vi "load_external_coordinates_grMD.vi"() -> ()   [LabVIEW 2017]
doc: "SciScan 1.2 160622"
uses:
  GFG/GFGDisplayRefsGet.vi
  GFG/GFGfpRefGet.vi
  GFG/GFGImageRefsGet.vi
  <vilib>/Utility/file.llb/Read From Spreadsheet File (I64).vi
  GFG/GFG library.lvlib
panel:
  out "error out":errorcluster
  in  "error in (no error)":errorcluster
  in  "stop":bool
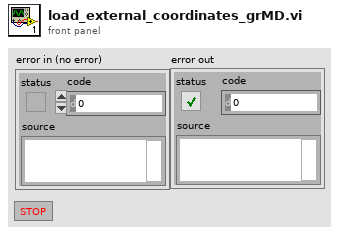
[diagram p1: front panel]
types:
  T1 = cluster{"Channel 1 small":refnum<vi>, "Channel 2 small":refnum<vi>, "Channel 3 small":refnum<vi>, "Channel 4 small":refnum<vi>, "Channel 1 large":refnum<vi>, "Channel 2 large":refnum<vi>, "Channel 3 large":refnum<vi>, "Channel 4 large":refnum<vi>, "RGB overlay":refnum<vi>, "ROI Image display":refnum<vi>, "arb line scan display":refnum<vi>, "Channel 5 large":refnum<vi>}
  T2 = typedef "IMAQ Image.ctl" = refnum<image>
  T3 = cluster{"Channel 1 small":T2, "Channel 2 small":T2, "Channel 3 small":T2, "Channel 4 small":T2, "Channel 1 large":T2, "Channel 2 large":T2, "Channel 3 large":T2, "Channel 4 large":T2, "RGB overlay":T2, "ROI Image display":T2, "arb line scan display":T2, "Channel 5 large":T2}
  T4 = cluster{"Contour Type":u32, "ROI Type":u32, i32[]}
  T5 = cluster{"Contour Type":u32, "ROI Type":u32, i32[]}[]
  T6 = cluster{i32[], cluster{"Contour Type":u32, "ROI Type":u32, i32[]}[]}
  T7 = cluster{"WaveformChartRef":refnum<vi>, "DigitalRef":refnum<vi>, "ArrayRef":refnum<vi>, "TabControlRef":refnum<vi>, "EnumRef":refnum<vi>, "RingRef":refnum<vi>, "BooleanRef":refnum<vi>, "KnobRef":refnum<vi>, "SlideRef":refnum<vi>, "PathRef":refnum<vi>, "StringRef":refnum<vi>, "ComboBox":refnum<vi>, "WaveformGraphRef":refnum<vi>}
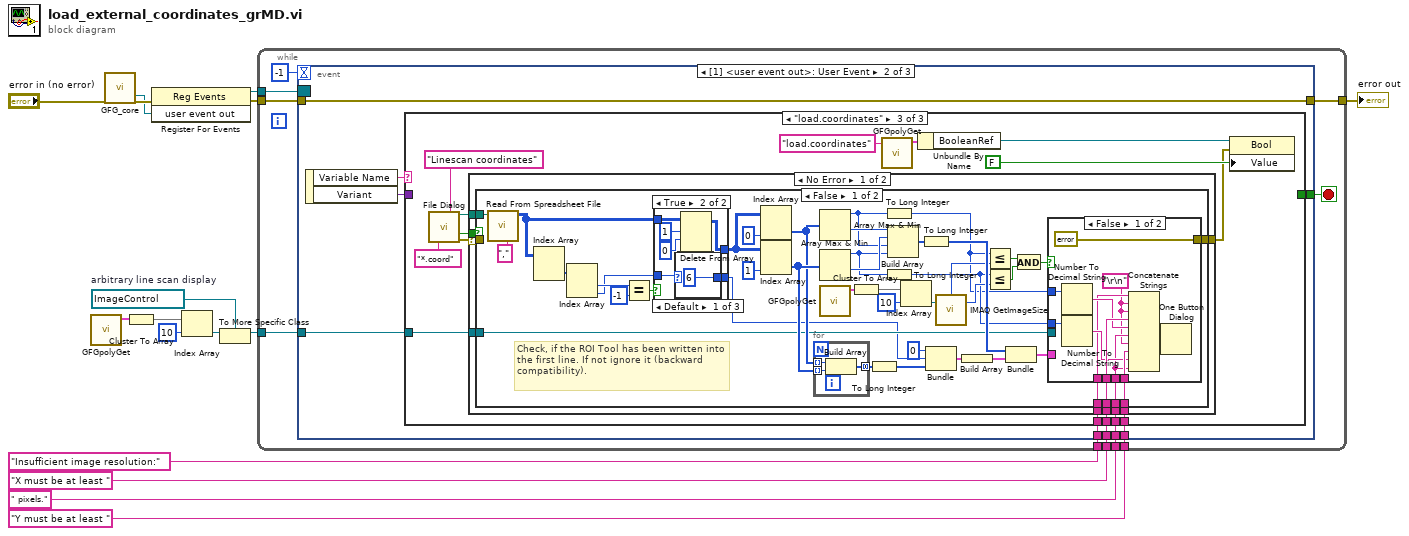
[diagram p0: block diagram]
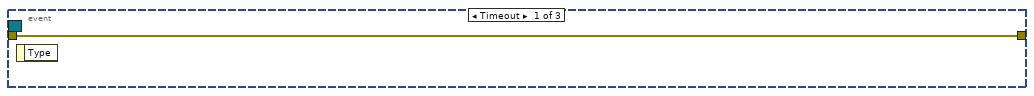
[diagram p2: hidden frame]
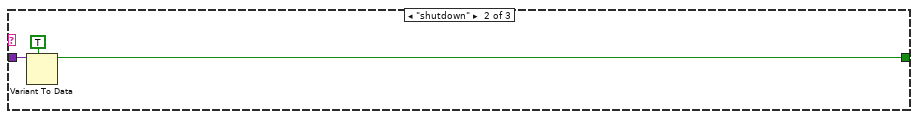
[diagram p4: hidden frame]
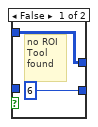
[diagram p5: hidden frame]
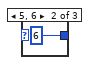
[diagram p6: hidden frame]
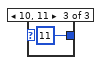
[diagram p7: hidden frame]
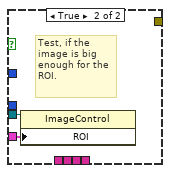
[diagram p8: hidden frame]
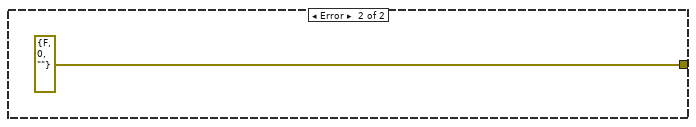
[diagram p10: hidden frame]
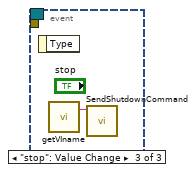
[diagram p11: hidden frame]
diagram:
  w16 = refnum<vi> refnum  # arbitrary line scan display
  n1 = call-poly "GFGpolyGet.vi"() -> ("DisplayRefsOut(generic class)"=w15:T1)  [unwired: 10 in, 1 out]
  n2 = call "GFG_core.vi"("error in (no error)"="error in (no error)") -> ("user event out"=w10:refnum<user-event>, "error out"=w11:errorcluster)  [unwired: 12 in, 5 out]
  n3 = Cluster To Array(cluster=w15) -> (array=w7:refnum<vi>[])
  n4 = register-events(error in=w11, w10) -> (reference out=w9:refnum<event-registration>, error out=w13:errorcluster)  [unwired: 1 in]
  n5 = Index Array(array=w7, index=10) -> (element=w5:refnum<vi>)
  n6 = To More Specific Class(target class=w16, reference=w5) -> (specific class reference=w8:refnum<vi>)  [unwired: 1 in, 1 out]
  n7 = while {
    tunnel: w9 -> [w26]
    tunnel: w13 -> [w24]
    tunnel: [w23] -> w14
    tunnel: w8 -> [w21]
    tunnel: "Insufficient image resolution:" ("message") -> [w20]
    tunnel: "X must be at least " ("message") -> [w19]
    tunnel: " pixels." ("message") -> [w18]
    tunnel: "Y must be at least " ("message") -> [w17]
    stop <- w25 stop-if-true
    n8 = event shown="[1] <user event out>: User Event" {
      selector: w26 -> [_ _ _]
      dyn-events: _ -> [_ _ _]
      timeout: -1 -> [_ _ _]
      tunnel: [_ w35 _] -> w25
      tunnel: w24 -> [w27 w34 _]
      tunnel: [w27 w34 _] -> w23
      tunnel: w21 -> [_ w33 _]
      tunnel: w20 -> [_ w31 _]
      tunnel: w19 -> [_ w30 _]
      tunnel: w18 -> [_ w29 _]
      tunnel: w17 -> [_ w28 _]
      event Timeout {
        n9 = event-data() -> ()  [unwired: 1 in, 1 out]
      }
      event User Event {
        n10 = event-data() -> ("Variable Name"=w36:string, "Variant"=w32:variant)  [unwired: 1 in]
        n11 = case shown="\"load.coordinates\"" w36 {
          tunnel: w32 -> [_ w39 _]
          tunnel: [_ w37 _] -> w35
          tunnel: w33 -> [_ _ w54]
          tunnel: w31 -> [_ _ w43]
          tunnel: w30 -> [_ _ w42]
          tunnel: w29 -> [_ _ w41]
          tunnel: w28 -> [_ _ w40]
          frame Default {
          }
          frame "shutdown" {
            n12 = Variant To Data(type=TRUE ("want seconds? (F)"), Variant=w39) -> (data=w37:bool)  [unwired: 1 in, 1 out]
          }
          frame "load.coordinates" {
            n13 = call "File Dialog"("pattern (all files)"="*.coord", "pattern label"="Linescan coordinates" ("pattern (all files)")) -> ("selected path"=w53:path, "cancelled"=w46:bool, "error out"=w52:errorcluster)  [unwired: 10 in, 1 out]
            n14 = case shown="No Error" w52 {
              selector: w52 -> [w60 _]
              tunnel: w54 -> [w63 _]
              tunnel: w53 -> [w62 _]
              tunnel: w46 -> [w61 _]
              tunnel: [w59 errorcluster {"status"=FALSE, "code"=0, "source"=""} ("error out")] -> w45
              tunnel: w43 -> [w58 _]
              tunnel: w42 -> [w57 _]
              tunnel: w41 -> [w56 _]
              tunnel: w40 -> [w55 _]
              frame No Error {
                n15 = case shown="False" w61 {
                  tunnel: w63 -> [w91 _]
                  tunnel: w62 -> [w90 _]
                  tunnel: w60 -> [_ _]
                  tunnel: [w81 _] -> w59
                  tunnel: w58 -> [w75 _]
                  tunnel: w57 -> [w74 _]
                  tunnel: w56 -> [w73 _]
                  tunnel: w55 -> [w72 _]
                  frame False {
                    # "Check, if the ROI Tool has been written into the first line. If not ignore it (backward compatibility)."
                    n16 = call-poly <vilib>:"Read From Spreadsheet File.vi"("delimiter (\\t)"="," ("delimiter (\\t)"), "file path (dialog if empty)"=w90) -> ("all rows"=w65:i64[][])  [unwired: 5 in, 4 out]
                    n17 = Index Array(array=w65) -> (element=w71:i64[])  [unwired: 2 in]
                    n18 = Index Array(array=w71) -> (element #1=w70:i64, element #2=w66:i64)  [unwired: 2 in]
                    n19 = Equal?(x=w70, y=i64 -1) -> (x = y?=w68:bool)
                    n20 = case shown="True" w68 {
                      tunnel: [u32 6 ("ROI Type") w113] -> w67
                      tunnel: w66 -> [_ w114]
                      tunnel: w65 -> [w107 w112]
                      tunnel: [w107 w111] -> w64
                      frame False {
                        # "no ROI Tool  found"
                      }
                      frame True {
                        n21 = case shown="Default" w114 {
                          tunnel: [u32 6 ("ROI Type") u32 6 ("ROI Type") u32 11 ("ROI Type")] -> w113
                          frame Default {
                          }
                          frame 5, 6 {
                          }
                          frame 10, 11 {
                          }
                        }
                        n22 = Delete From Array(array=w112, length=1, index (row)=0) -> (array with subset deleted=w111:i64[][])  [unwired: 1 in, 1 out]
                      }
                    }
                    n23 = Index Array(array=w64, index (col)=0 ("disabled index (col)")) -> (element=w99:i64[])  [unwired: 1 in]
                    n24 = Index Array(array=w64, index (col)=1 ("disabled index (col)")) -> (element=w100:i64[])  [unwired: 1 in]
                    n25 = for {
                      tunnel: w99 -> [w133] mode=indexing
                      tunnel: w100 -> [w132] mode=indexing
                      tunnel: [w131] -> w102 mode=concatenating
                      n26 = Build Array(w133, w132) -> (w131:i64[])
                    }
                    n27 = Array Max & Min(array=w99) -> (max value=w80:i64, min value=w96:i64)  [unwired: 2 out]
                    n28 = Array Max & Min(array=w100) -> (max value=w79:i64, min value=w97:i64)  [unwired: 2 out]
                    n29 = call-poly "GFGpolyGet.vi"() -> ("Image Refs Out"=w86:T3)  [unwired: 10 in, 1 out]
                    n30 = Cluster To Array(cluster=w86) -> (array=w88:T2[])
                    n31 = To Long Integer(number=w102) -> (32bit integer=w103:i32[])
                    n32 = To Long Integer(number=w80) -> (32bit integer=w76:i32)
                    n33 = To Long Integer(number=w79) -> (32bit integer=w77:i32)
                    n34 = Build Array(w96, w97, w80, w79) -> (w98:i64[])
                    n35 = Index Array(array=w88, index=10) -> (element=w89:T2)
                    n36 = To Long Integer(number=w98) -> (32bit integer=w106:i32[])
                    n37 = Bundle("Contour Type"=u32 0, "ROI Type"=w67, w103) -> (w104:T4)  [unwired: 1 in]
                    n38 = call "IMAQ GetImageSize"("Image"=w89) -> ("Y Resolution"=w78:i32, "X Resolution"=w85:i32)  [unwired: 3 in, 1 out]
                    n39 = Build Array(w104) -> (w105:T5)
                    n40 = Less Or Equal?(x=w76, y=w85) -> (x <= y?=w84:bool)
                    n41 = Less Or Equal?(x=w77, y=w78) -> (x <= y?=w83:bool)
                    n42 = Bundle(w106, w105) -> (w92:T6)  [unwired: 1 in]
                    n43 = And(x=w84, y=w83) -> (x .and. y?=w82:bool)
                    n44 = case shown="False" w82 {
                      tunnel: w92 -> [_ w130]
                      tunnel: w91 -> [_ w129]
                      tunnel: [errorcluster {"status"=FALSE, "code"=0, "source"=""} ("error out") _] -> w81
                      tunnel: w77 -> [w126 _]
                      tunnel: w76 -> [w127 _]
                      tunnel: w75 -> [w119 _]
                      tunnel: w74 -> [w124 _]
                      tunnel: w73 -> [w120 _]
                      tunnel: w72 -> [w122 _]
                      frame False {
                        w118 = "\r\n"
                        n45 = Number To Decimal String(number=w127) -> (decimal integer string=w123:string)  [unwired: 1 in]
                        n46 = Number To Decimal String(number=w126) -> (decimal integer string=w121:string)  [unwired: 1 in]
                        n47 = Concatenate Strings(w119, w118, w118, w124, w123, w120, w118, w122, w121, w120) -> (w125:string)
                        n48 = One Button Dialog(message=w125) -> ()  [unwired: 1 in, 1 out]
                      }
                      frame True {
                        # "Test, if the image is big enough for the ROI."
                        n49 = property class="ImageControl"(reference=w129, "ROI"=w130) -> ()  [unwired: 1 in, 2 out]
                      }
                    }
                  }
                  frame True {
                  }
                }
              }
              frame Error {
              }
            }
            n50 = call-poly "GFGpolyGet.vi"("Variable Name in"="load.coordinates") -> ("output cluster"=w50:T7)  [unwired: 9 in, 1 out]
            n51 = Unbundle By Name(w50) -> ("BooleanRef"=w49:refnum<vi>)
            n52 = property class="Bool"(reference=w49, error in=w45, "Value"=FALSE) -> ()  [unwired: 2 out]
          }
        }
      }
      event "stop": Value Change {
        n53 = event-data() -> ()  [unwired: 1 in, 1 out]
        n54 = call "getVIname.vi"() -> ("VI name"=w135:string)  [unwired: 19 in]
        n55 = call "SendShutdownCommand.vi"("Source VI"=w135) -> ()  [unwired: 11 in]
      }
    }
  }
  "error out" <- w14
